vi "Wait for Prompt.vi"(8 "error in (no error)":errorcluster, 10 "Retries (5)":i32=5, 11 "Controller States in":T1) -> (0 "error out":errorcluster, 2 "Found Cue?":bool, 3 "Controller States out":T1)   [LabVIEW 2019, in "Controller.lvlib"]
uses:
  Controller.lvlib
  Controller States.ctl
  <vilib>/ErrorRing/Error Ring.xnode
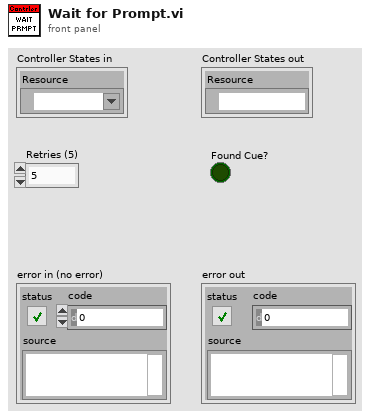
[diagram p1: front panel]
types:
  T1 = typedef "Controller.lvlib/Controller States.ctl" = cluster{"Resource":refnum<visa-resource-name>}
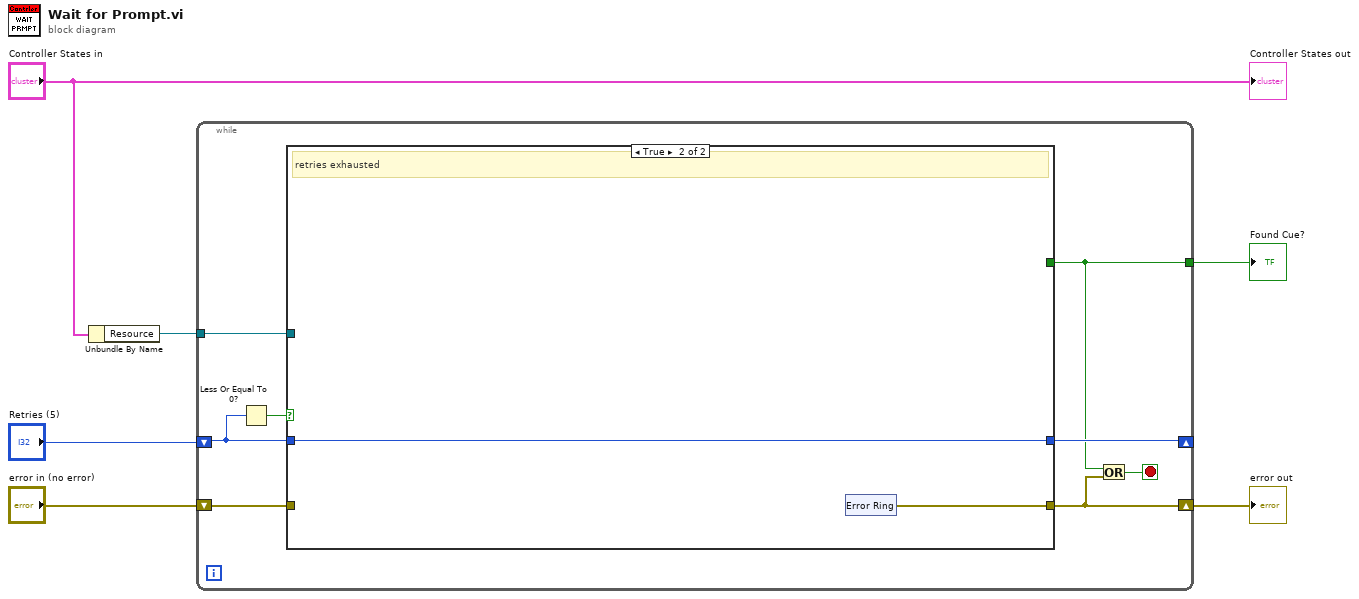
[diagram p0: block diagram]
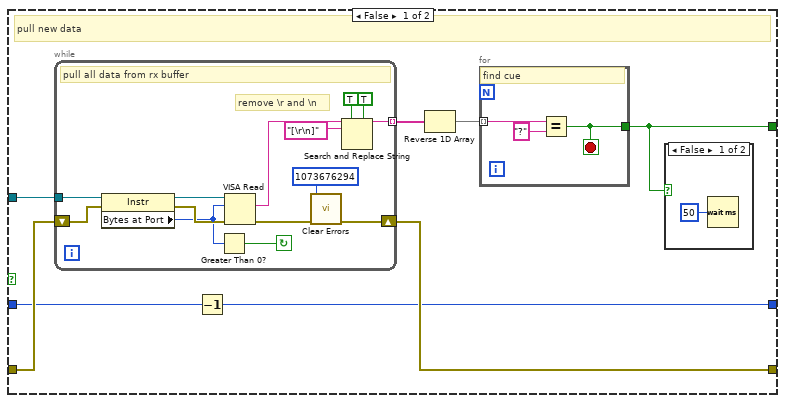
[diagram p2: hidden frame]
diagram:
  n1 = Unbundle By Name("Controller States in") -> ("Resource"=w3:refnum<visa-resource-name>)
  n2 = while {
    tunnel: w3 -> [w14]
    shift-right: [w8] -> w5
    shift-left: "error in (no error)" -> [w13]
    shift-right: [w10] -> _
    shift-left: "Retries (5)" -> [w11]
    tunnel: [w7] -> w1
    stop <- w9 stop-if-true
    n3 = Less Or Equal To 0?(x=w11) -> (x <= 0?=w12:bool)
    n4 = case shown="True" w12 {
      tunnel: w14 -> [w22 _]
      tunnel: w13 -> [w21 _]
      tunnel: w11 -> [w17 w42]
      tunnel: [w20 w41] -> w8
      tunnel: [w15 _] -> w7
      tunnel: [w16 w42] -> w10
      frame False {
        # "pull new data"
        n5 = while {
          tunnel: w22 -> [w40]
          shift-right: [w33] -> w20
          shift-left: w21 -> [w38]
          tunnel: [w27] -> w19 mode=indexing
          stop <- w34 continue-if-true
          # "remove \\r and \\n"
          # "pull all data from rx buffer"
          n6 = property class="Instr"(reference=w40, error in=w38) -> (reference out=w39:refnum<visa-resource-name>, error out=w37:errorcluster, "Bytes at Port"=w35:u32)
          n7 = Greater Than 0?(x=w35) -> (x > 0?=w34:bool)
          n8 = VISA Read(VISA resource name=w39, byte count=w35, error in (no error)=w37) -> (read buffer=w31:string, error out=w36:errorcluster)  [unwired: 2 out]
          n9 = call <vilib>:"Clear Errors.vi"("error in (no error)"=w36, "specific error code to clear (0: all)"=1073676294 ("Code")) -> ("error out"=w33:errorcluster)  [unwired: 4 in, 1 out]
          n10 = Search and Replace String(replace all?=TRUE ("replace all? (F)"), multiline?=TRUE ("multiline? (F)"), input string=w31, search string="[\r\n]") -> (result string=w27:string)  [unwired: 4 in, 3 out]
        }
        n11 = Decrement(x=w17) -> (x-1=w16:i32)
        n12 = Reverse 1D Array(array=w19) -> (reversed array=w18:string[])
        n13 = for {
          tunnel: w18 -> [w26] mode=indexing
          tunnel: [w24] -> w15
          stop <- w24 stop-if-true
          # "find cue"
          n14 = Equal?(x=w26, y="?") -> (x = y?=w24:bool)
        }
        n15 = case shown="False" w15 {
          frame False {
            n16 = Wait (ms)(milliseconds to wait=u32 50) -> ()  [unwired: 1 out]
          }
          frame True {
          }
        }
      }
      frame True {
        # "retries exhausted"
        n17 = xnode "Error Ring"() -> ("error out"=w41:errorcluster)
      }
    }
    n18 = Or(x=w7, y=w8) -> (x .or. y?=w9:bool)
  }
  "error out" <- w5
  "Found Cue?" <- w1
  "Controller States out" <- "Controller States in"
